vi "Insert Front Panel.vi"(8 "error in (no error)":errorcluster, 9 "Insertion Request Time":timestamp, 10 "Protected Subpanel":T1, 11 "ViewableChart in":refnum<class "ViewableChart.lvclass">) -> (0 "error out":errorcluster, 3 "ViewableChart out":refnum<class "ViewableChart.lvclass">)   [LabVIEW 2017, in "ViewableChart.lvclass"]
doc: "<License>\nCopyright © 2017 Composed Systems, LLC | All rights reserved\nwww.composed.io\n\nAuthor: Ethan Stern <ethan.stern@composed.io>\n\nThis software is provided \"AS IS\" WITHOUT WARRANTIES, either express or implied, AND IS FOR EDUCATIONAL PURPOSES ONLY.\n</License>MVA Framework 1.7.0.33\nEthan Stern - Composed Systems\nCopyright (c) 2018, Composed Systems"
uses:
  ViewableChart.lvclass
  mva-viewable/Source/IViewable/ProtectedSubpanel/Protected Subpanel Reference.ctl
  mva-viewable/Source/IViewable/ProtectedSubpanel/ProtectedSubpanel.lvclass
  ViewableChart.lvclass/ViewableChart.ctl
  mva-viewable/Source/IViewable/IViewable/IViewable.lvclass
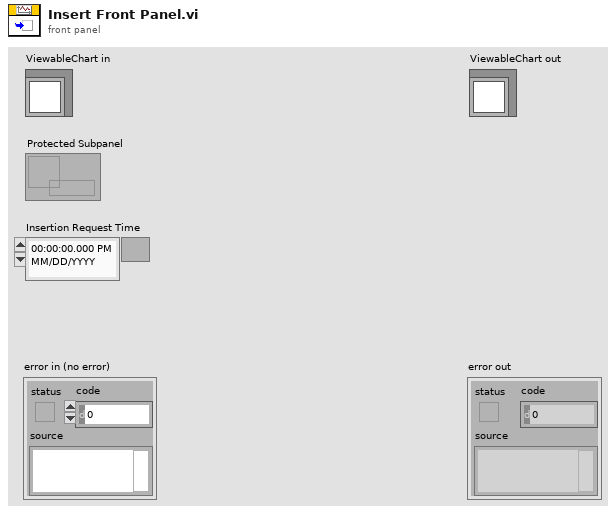
[diagram p1: front panel]
types:
  T1 = typedef "IViewable.lvlib/ProtectedSubpanel.lvclass/Protected Subpanel Reference.ctl" = refnum<data-value>
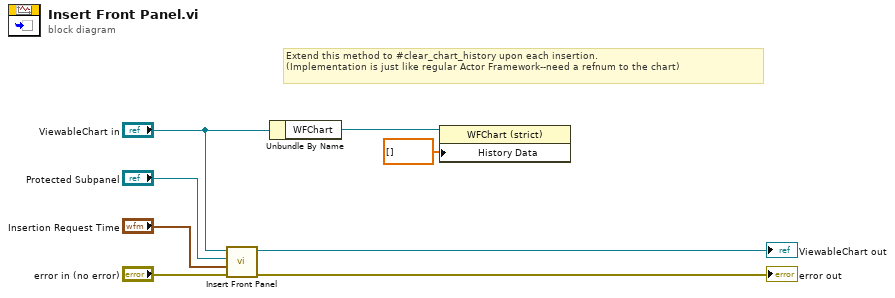
[diagram p0: block diagram]
diagram:
  # "Extend this method to #clear_chart_history upon each insertion.\n(Implementation is just like regular Actor Framework--need a refnum to the chart)"
  n1 = call-parent "Insert Front Panel.vi"("error in (no error)"="error in (no error)", "Insertion Request Time"="Insertion Request Time", "Protected Subpanel"="Protected Subpanel", "IViewable in"="ViewableChart in") -> ("error out"=→"error out":errorcluster, "IViewable out"=→"ViewableChart out":refnum<class "ViewableChart.lvclass">)  [unwired: 6 in]
  n2 = Unbundle By Name("ViewableChart in") -> ("WFChart"=w2:refnum<vi>)
  n3 = property class="WFChart (strict)"(reference=w2, "History Data"=dbl[] []) -> ()  [unwired: 1 in, 2 out]
